vi "epoch access point to epoch microsecond.vi"(10 "dest":cluster{}, 11 "sync_value":cluster{}) -> (2 "dest out":cluster{}, 3 "function return":i32)   [LabVIEW 2019, in "apdm.lvlib"]
doc: "APDM_EXPORT int apdm_epoch_access_point_to_epoch_microsecond(const uint64_t sync_value, struct timeval *dest);"
uses:
  apdm.lvlib
  Lee Lab/CP FES Walking 2018/Code/Working/LabVIEW/apdm.dll
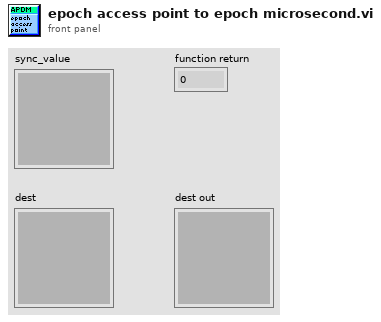
[diagram p1: front panel]
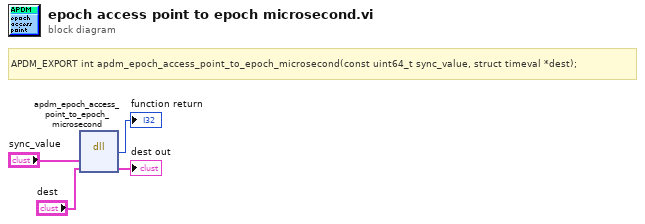
[diagram p0: block diagram]
diagram:
  # "APDM_EXPORT int apdm_epoch_access_point_to_epoch_microsecond(const uint64_t sync_value, struct timeval *dest);"
  n1 = dll-call lib="C:/Users/jfalesi/Dropbox/Lee Lab/CP FES Walking 2018/Code/Working/LabVIEW/apdm.*" fn="apdm_epoch_access_point_to_epoch_microsecond"("sync_value"="sync_value", "dest"="dest") -> (→"function return":i32, "dest"=→"dest out":cluster{})  [unwired: 4 in, 2 out]
